vi "wrap.PullVariantString.vi"(0 "class.GLue in":refnum<class "class.GLue.lvclass">, 11 "error in (no error)":errorcluster, 13 "Index":i32=-1) -> (4 "class.GLue out":refnum<class "class.GLue.lvclass">, 6 "VarString":string, 10 "Return":i32, 15 "error out":errorcluster)   [LabVIEW 2014, in "GLue.lvlib" / "class.GLue.lvclass"]
uses:
  class.GLue.lvclass
  class.GLue.lvclass/class.GLue.ctl
  Resources/GLue.dll
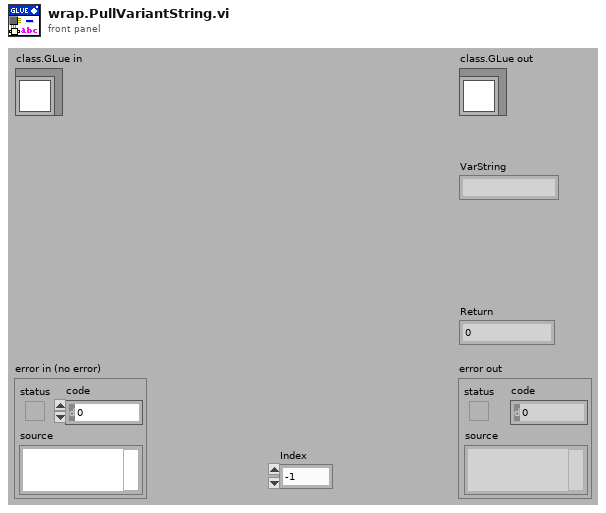
[diagram p1: front panel]
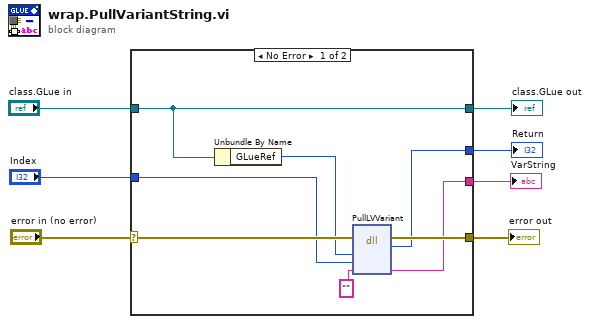
[diagram p0: block diagram]
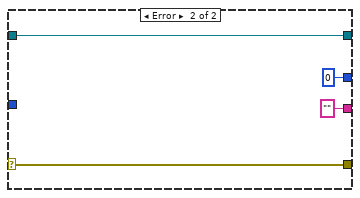
[diagram p2: hidden frame]
diagram:
  n1 = case shown="No Error" "error in (no error)" {
    selector: "error in (no error)" -> [w14 w19]
    tunnel: [w13 w19] -> w6
    tunnel: [w15 w18] -> w4
    tunnel: "class.GLue in" -> [w15 w18]
    tunnel: "Index" -> [w11 _]
    tunnel: [w10 "" ("String")] -> w2
    tunnel: [w8 0 ("return type")] -> w1
    frame No Error {
      n2 = Unbundle By Name(w15) -> ("GLueRef"=w12:i64)
      n3 = dll-call lib="C:/Users/Antonie/Documents/work/glue/trunk/Resources/GLue.dll" fn="PullLVVariant"(error in=w14, "MLua"=w12, "Index"=w11, "VarString"="" ("String")) -> (error out=w13:errorcluster, "return type"=w8:i32, "VarString"=w10:string)  [unwired: 4 in, 1 out]
    }
    frame Error {
    }
  }
  "error out" <- w6
  "class.GLue out" <- w4
  "VarString" <- w2
  "Return" <- w1
